vi "Tank Simulation_DS.vi"() -> ()   [LabVIEW 2009]
doc: "Tank Simulation displays a history of inflow, level, and temperature in a simulated tank control application. This example has been modified from the sample application suppiled by LabVIEW. The modification are to support application control and data logging using an iLabs Interactive LabServer.\n\n1. The 'Power' control has been renamed to stop, default set to False and loop termination changed to 'stop when true'. The VI's 'stop' control is set to true when a reservation has expired. The VI should clean-up and end execution when 'stop' is true.\n\n2. DataSocket is used to write a single cluster of data values to dstp://localhost/TankSim.dat each loop. The data is encoded as XML. If the DataSocket is specified in the application's information in the labserver the data will be stored on the ESS with the current experimentID."
panel:
  in  "Low Temp Limit (deg F)":dbl=95.0 format="%0.2f"
  in  "High Temp Limit (deg F)":dbl=105.0 format="%0.2f"
  in  "Low Level Limit (lbm)":dbl=0.3 format="%0.2f"
  in  "High Level Limit (lbm)":dbl=0.7 format="%0.2f"
  in  "Heat Inflow Rate (lbm.T/s)":dbl=19.0 format="%0.2f"
  in  "Time/Sim Cycle (min)":dbl=0.1 format="%0.2f"
  in  "Inlet Temp (deg F)":dbl=67.7 format="%0.2f"
  in  "Inflow Rate (lbm/min)":dbl=0.55 format="%0.2f"
  in  "Tank Temp (deg F)":dbl=70.0 format="%0.2f"
  in  "Tank Level (ft)":dbl=0.5000038146972656 format="%0.2f"
  out "?":bool=TRUE
  out "deg F":dbl=64.00073008107321 format="%0.2f"
  out "lbm/min":dbl=-0.06250076915563287 format="%0.2f"
  out "lbm":dbl=0.5000046618394537 format="%0.2f"
  out "Tank Level History":dbl(graph)
  out "Inflow Rate History":dbl(graph)
  out "Tank Temperature History":dbl(graph)
  in  "stop":bool caption="Power"
  out "Elapsed Tme (sec)":dbl=4.000057983398437 format="%0.2f"
  out "Current Level (ft)":dbl(slide)=0.5000046618394537 scale=0.0..1.0000000000000002 scale format="%0.2f"
  out "?":bool=TRUE
  # "Inflow Rate History"
  # "Tank Level History"
  # "Tank Temperature History"
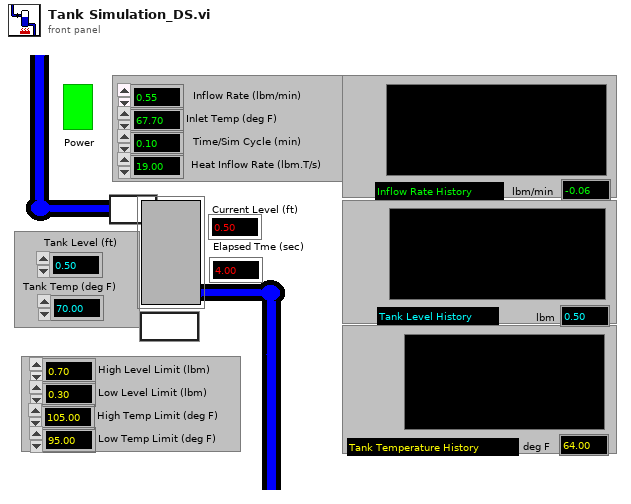
[diagram p1: front panel]
types:
  T1 = enum16{"Read", "Write", "ReadWrite", "BufferedRead", "BufferedReadWrite"}
  T2 = cluster{"Time/Sim Cycle (min)":dbl, dbl, dbl, "New Level":dbl, "New Temp":dbl}
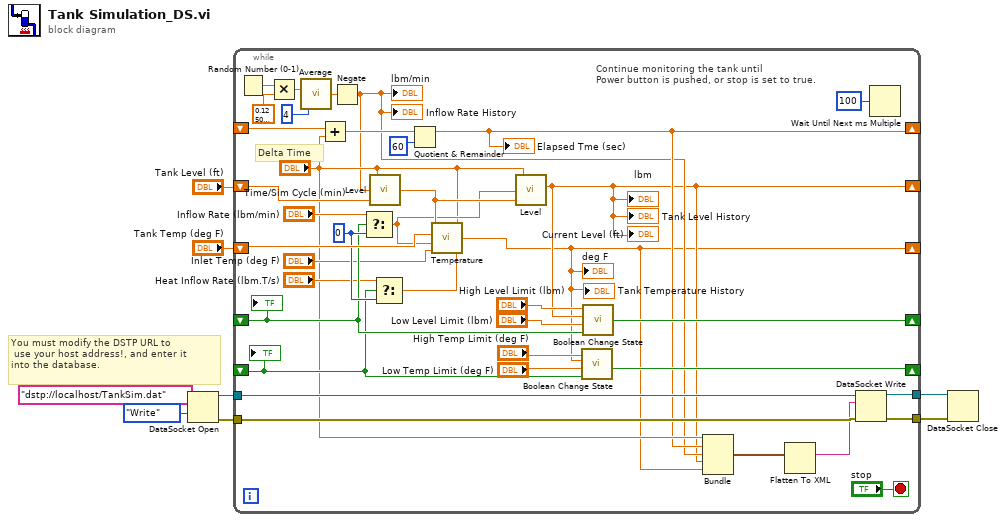
[diagram p0: block diagram]
diagram:
  # "You must modify the DSTP URL to\n use your host address!, and enter it\ninto the database."
  n1 = DataSocket Open(10:T1."Write" ("mode"), 11:"dstp://localhost/TankSim.dat" ("URL")) -> (0:w2:errorcluster, 3:w4:refnum<k13>)  [unwired: 2 in]
  n2 = while {
    shift-left: _ -> [w44]
    shift-right: [w14] -> _
    shift-left: "Tank Level (ft)" -> [w35]
    shift-right: [w12] -> _
    shift-left: "Tank Temp (deg F)" -> [w38]
    shift-right: [w11] -> _
    shift-left: _ -> [w31]
    shift-right: [w39] -> _
    shift-left: _ -> [w32]
    shift-right: [w40] -> _
    tunnel: w4 -> [w19]
    tunnel: [w18] -> w3
    tunnel: w2 -> [w17]
    tunnel: [w16] -> w1
    stop <- "stop" stop-if-true
    w37 = 0
    # "Continue monitoring the tank until\nPower button is pushed, or stop is set to true."
    # "Delta Time"
    n3 = Random Number (0-1)() -> (number: 0 to 1=w30:dbl)
    n4 = Multiply(x=w30, y=0.12500152587890626) -> (x*y=w28:dbl)
    n5 = call "Average.vi"("Queue Size"=4, "New Value"=w28) -> ("Waveform Chart"=w45:dbl)
    n6 = Add(x=w44, y="Time/Sim Cycle (min)") -> (x+y=w42:dbl)
    n7 = Negate(x=w45) -> (-x=w13:dbl)
    "lbm/min" <- w13
    "Inflow Rate History" <- w13
    n8 = Select(t="Inflow Rate (lbm/min)", s=w32, f=w37) -> (s? t:f=w34:dbl)
    n9 = call "Level.vi"("Initail Level"=w35, "Mass Flow Rate"=w13, "Elapsed Time"="Time/Sim Cycle (min)") -> ("New Level"=w41:dbl)
    n10 = Select(t="Heat Inflow Rate (lbm.T/s)", s=w31, f=w37) -> (s? t:f=w36:dbl)
    n11 = Quotient & Remainder(x=w42, y=60) -> (x-y*floor(x/y)=w14:dbl)  [unwired: 1 out]
    "Elapsed Tme (sec)" <- w14
    n12 = call "Temperature.vi"("Heat Flow Rate"=w36, "Elapsed Time"="Time/Sim Cycle (min)", "Inlet Fluid Temp"="Inlet Temp (deg F)", "Inlet Mass Flow Rate"=w34, "Initial Fluid Temp"=w38, "Initial Fluid Mass"=w41) -> ("New Temp"=w11:dbl)
    "deg F" <- w11
    "Tank Temperature History" <- w11
    n13 = call "Level.vi"("Initail Level"=w41, "Mass Flow Rate"=w34, "Elapsed Time"="Time/Sim Cycle (min)") -> ("New Level"=w12:dbl)
    "lbm" <- w12
    "Current Level (ft)" <- w12
    "Tank Level History" <- w12
    n14 = call "Boolean Change State.vi"("Current State"=w31, "Low Limit"="Low Temp Limit (deg F)", "Current Value"=w11, "High Limit"="High Temp Limit (deg F)") -> ("New State"=w39:bool)
    n15 = call "Boolean Change State.vi"("Current State"=w32, "Low Limit"="Low Level Limit (lbm)", "Current Value"=w12, "High Limit"="High Level Limit (lbm)") -> ("New State"=w40:bool)
    n16 = Bundle("Time/Sim Cycle (min)"="Time/Sim Cycle (min)", w14, w13, "New Level"=w12, "New Temp"=w11) -> (w10:T2)  [unwired: 1 in]
    n17 = Flatten To XML(anything=w10) -> (xml string=w9:string)
    n18 = DataSocket Write(8:w17, 10:w9, 11:w19) -> (0:w16:errorcluster, 3:w18:refnum<k13>)  [unwired: 1 in, 1 out]
    n19 = Wait Until Next ms Multiple(millisecond multiple=u32 100) -> ()  [unwired: 1 out]
    "?" <- w32
    "?" <- w31
  }
  n20 = DataSocket Close(8:w1, 11:w3) -> ()  [unwired: 1 in, 2 out]
